vi "Move.vi"(7 "VI":refnum<vi>, 8 "Error":errorcluster, 11 "(FPPos)":refnum<class "Frame_FPPos.lvclass">) -> (0 "Error Out":errorcluster, 3 "(FPPos) Out":refnum<class "Frame_FPPos.lvclass">, 5 "VI Out":refnum<vi>)   [LabVIEW 2025, in "Frame_FPPos.lvclass"]
uses:
  Frame_FPPos.lvclass
  Frame_FPPos.lvclass/Frame_FPPos.ctl
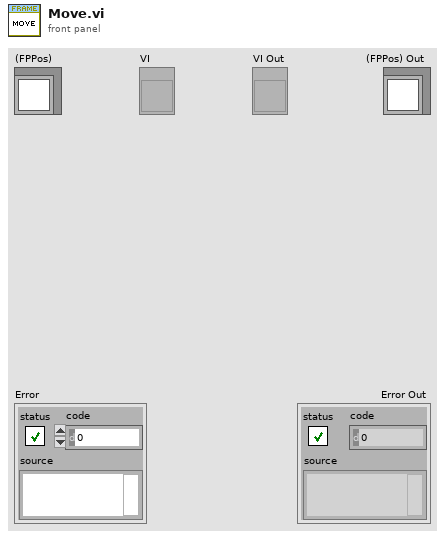
[diagram p1: front panel]
types:
  T1 = typedef "LVRectTypeDef.ctl" = cluster{"Left":i16, "Top":i16, "Right":i16, "Bottom":i16}
  T2 = typedef "ENUM RB_Pos_Quadrant Position.ctl" = enum32{"LFT-TOP", "MID-TOP", "RGT-TOP", "LFT-CTR", "MID-CTR", "RGT-CTR", "LFT-BOT", "MID-BOT", "RGT-BOT"}
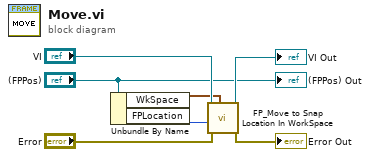
[diagram p0: block diagram]
diagram:
  n1 = Unbundle By Name("(FPPos)") -> ("WkSpace"=w2:T1, "FPLocation"=w1:T2)
  n2 = call "FP_Move to Snap Location In WorkSpace.vi"("WkSpace"=w2, "Error"="Error", "Snap Location"=w1, "VI"="VI") -> ("Error Out"=→"Error Out":errorcluster, "VI Out"=→"VI Out":refnum<vi>)  [unwired: 6 in]
  "(FPPos) Out" <- "(FPPos)"
